vi "StateSpaceEqn.vi"(5 "u":dbl, 7 "x":dbl[](array[numeric]) format="%.2f", 8 "D":dbl[](array[numeric]) format="%.2f", 9 "C":dbl[](array[numeric]) format="%.2f", 10 "B":dbl[](array[numeric]) format="%.2f", 11 "A":T1) -> (2 "y(t)":dbl[](array[numeric]), 3 "x(t+1)":dbl[](array[numeric]))   [LabVIEW 2018]
uses:
  <vilib>/Analysis/Matrix/Datatypes/RealMatrix.ctl
  <vilib>/Analysis/7linalg.llb/Solve Linear Equations (single right hand).vi
  <vilib>/Analysis/baseanly.llb/Solve Linear Equations By Cholesky.vi
  <vilib>/Analysis/baseanly.llb/Real Matrix to Compact Array.vi
  <vilib>/Analysis/baseanly.llb/Real Compact Tri-Matrix Linear Eqs.vi
  <vilib>/Analysis/7linalg.llb/Solve Linear Eqs (General).vi
  <vilib>/Analysis/7linalg.llb/Solve Linear Eqs (Gen, single right hand).vi
  <vilib>/Analysis/NI_AALPro.lvlib
  <vilib>/Analysis/Matrix/NI_Matrix.lvlib
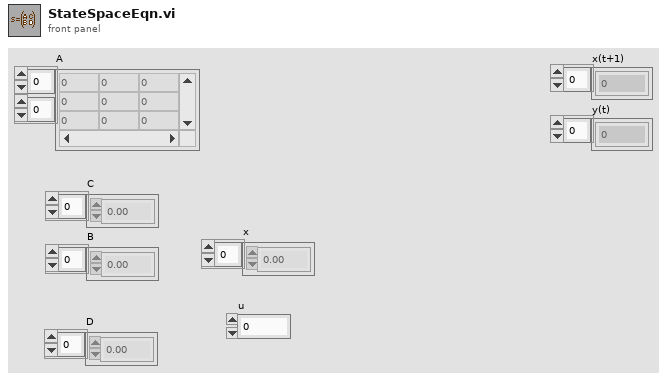
[diagram p1: front panel]
types:
  T1 = typedef "NI_Matrix.lvlib/RealMatrix.ctl" = dbl[][]
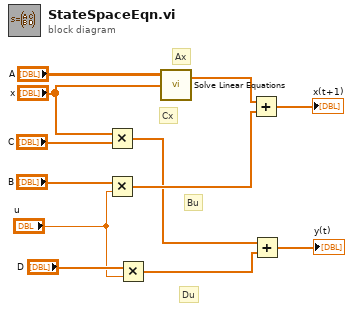
[diagram p0: block diagram]
diagram:
  # "Du"
  # "Cx"
  # "Bu"
  # "Ax"
  n1 = Multiply(x="x", y="C") -> (x*y=w2:dbl[])
  n2 = Multiply(x="B", y="u") -> (x*y=w7:dbl[])
  n3 = Multiply(x="D", y="u") -> (x*y=w3:dbl[])
  n4 = call-poly <vilib>:"Solve Linear Equations.vi"("Known Vector"="x", "Input Matrix"="A") -> ("Solution Vector"=w8:dbl[])  [unwired: 1 in, 1 out]
  n5 = Add(x=w8, y=w7) -> (x+y=→"x(t+1)":dbl[])
  n6 = Add(x=w2, y=w3) -> (x+y=→"y(t)":dbl[])
